vi "Write Rotator.vi"(8 "error in (no error)":errorcluster, 10 "Rotator":dbl, 11 "angles in":refnum<class "angles.lvclass">) -> (0 "error out":errorcluster, 3 "angles out":refnum<class "angles.lvclass">)   [LabVIEW 2018, in "angles.lvclass"]
uses:
  angles.lvclass
  angles.lvclass/angles.ctl
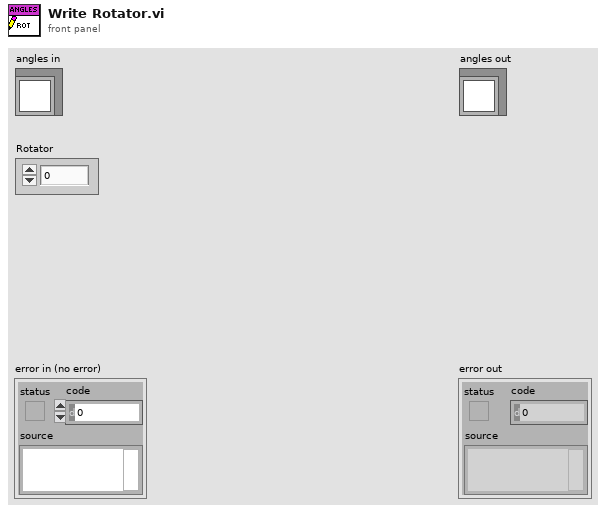
[diagram p1: front panel]
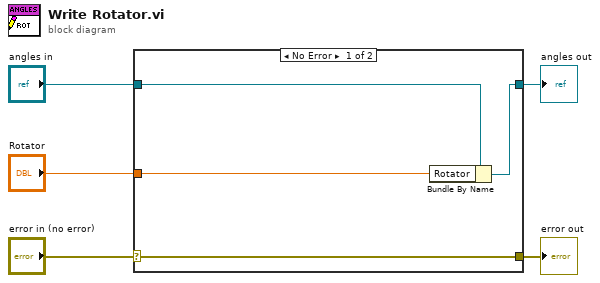
[diagram p0: block diagram]
diagram:
  n1 = case shown="No Error" "error in (no error)" {
    selector: "error in (no error)" -> [w9 w10]
    tunnel: [w9 w10] -> w4
    tunnel: [w7 w11] -> w2
    tunnel: "angles in" -> [w8 w11]
    tunnel: "Rotator" -> [w6 _]
    frame No Error {
      n2 = Bundle By Name(cluster=w8, "Rotator"=w6) -> (w7:refnum<class "angles.lvclass">)
    }
    frame Error {
    }
  }
  "error out" <- w4
  "angles out" <- w2
